vi "Eliminated.vi"(6 "Column":i32, 8 "Row":i32, 9 "Killer Index":i32, 10 "Team Index":i32, 11 "third in":refnum<class "third.lvclass">) -> (3 "third out":refnum<class "third.lvclass">)   [LabVIEW 2015, in "third.lvclass"]
uses:
  third.lvclass
  Square/Square.lvclass
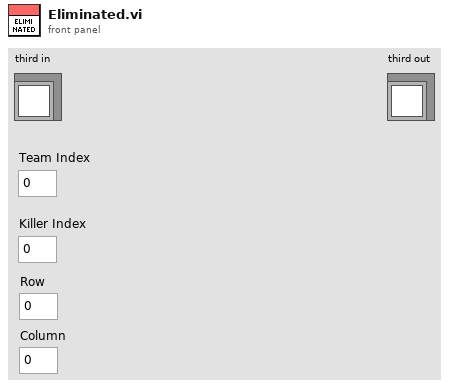
[diagram p1: front panel]
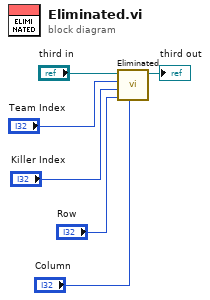
[diagram p0: block diagram]
diagram:
  n1 = call-parent "Eliminated.vi"("Column"="Column", "Row"="Row", "Killer Index"="Killer Index", "Team Index"="Team Index", "Square in"="third in") -> ("Square out"=→"third out":refnum<class "third.lvclass">)  [unwired: 6 in]
